vi "SaveOnFile1.vi"() -> ()   [LabVIEW 2019]
uses:
  <vilib>/Analysis/Matrix/Datatypes/RealMatrix.ctl
  <vilib>/Utility/file.llb/Write Delimited Spreadsheet (I64).vi
  <vilib>/Analysis/Matrix/NI_Matrix.lvlib
panel:
  out "2D matrix":T1
  in  "linhas":i32
  in  "colunas":i32
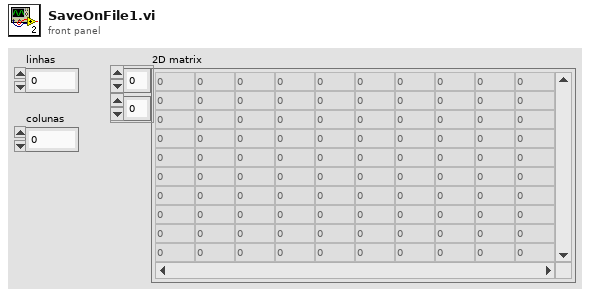
[diagram p1: front panel]
types:
  T1 = typedef "NI_Matrix.lvlib/RealMatrix.ctl" = dbl[][]
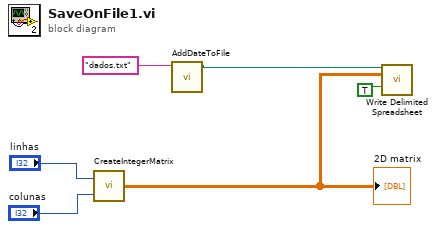
[diagram p0: block diagram]
diagram:
  n1 = call "CreateIntegerMatrix.vi"("colunas"="colunas", "linhas"="linhas") -> ("2D matrix"=w5:T1)
  "2D matrix" <- w5
  n2 = call "AddDateToFile.vi"("file name"="dados.txt") -> ("new file path (Not A Path if cancelled)"=w4:path)  [unwired: 9 in, 1 out]
  n3 = call-poly <vilib>:"Write Delimited Spreadsheet.vi"("file path (dialog if empty)"=w4, "2D data"=w5, "append to file? (new file:F)"=TRUE) -> ()  [unwired: 11 in, 2 out]
